vi "Unflatten I16.vi"(3 "Flat Data":u8[](array[numeric]) format="%.0x", 4 "Endian":T1) -> (5 "I16":i16)   [LabVIEW 2021, in "DataTypes_CIF_U.lvlib"]
uses:
  DataTypes_CIF_U.lvlib
  Typedef/Endian.ctl
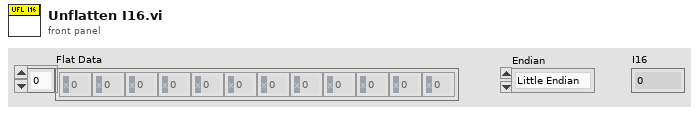
[diagram p1: front panel]
types:
  T1 = typedef "DataTypes_CIF_U.lvlib/Endian.ctl" = enum16{"Little Endian", "Big Endian"}
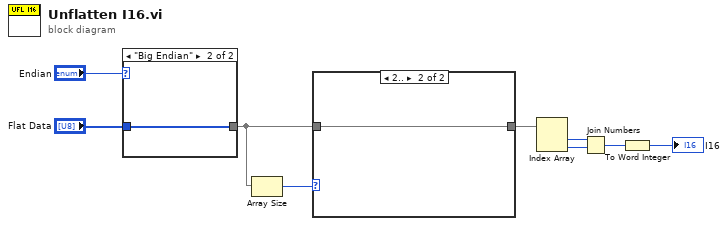
[diagram p0: block diagram]
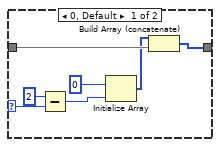
[diagram p2: hidden frame]
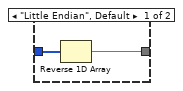
[diagram p3: hidden frame]
diagram:
  n1 = case shown="\"Big Endian\"" "Endian" {
    tunnel: "Flat Data" -> [w11 w12]
    tunnel: [w10 w12] -> w3
    frame "Little Endian", Default {
      n2 = Reverse 1D Array(array=w11) -> (reversed array=w10:u8[])
    }
    frame "Big Endian" {
    }
  }
  n3 = Array Size(array=w3) -> (size(s)=w6:i32)
  n4 = case shown="2.." w6 {
    selector: w6 -> [w19 _]
    tunnel: w3 -> [w15 w20]
    tunnel: [w13 w20] -> w4
    frame 0, Default {
      n5 = Subtract(x=2, y=w19) -> (x-y=w16:i32)
      n6 = Initialize Array(u8 0 ("element"), w16) -> (w14:u8[])
      n7 = Build Array (concatenate)(w14, w15) -> (w13:u8[])
    }
    frame 2.. {
    }
  }
  n8 = Index Array(array=w4) -> (element #1=w8:u8, element #2=w7:u8)  [unwired: 2 in]
  n9 = Join Numbers(hi=w8, lo=w7) -> ((hi.lo)=w1:u16)
  n10 = To Word Integer(number=w1) -> (16bit integer=→"I16":i16)
